vi "Read Numeric Text.vi"(9 "Digital in":refnum<class "Digital.lvclass">) -> (3 "Digital out":refnum<class "Digital.lvclass">, 4 "NumericText":refnum<class "NumericText.lvclass">)   [LabVIEW 2014, in "Raspberry Pi Compatible Compiler for LabVIEW.lvlib" / "Digital.lvclass"]
uses:
  Digital.lvclass
  NumericText/NumericText.lvclass
  Digital.lvclass/Digital.ctl
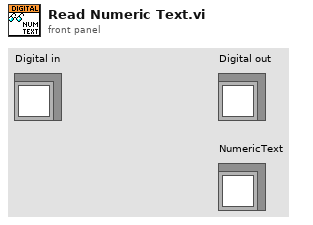
[diagram p1: front panel]
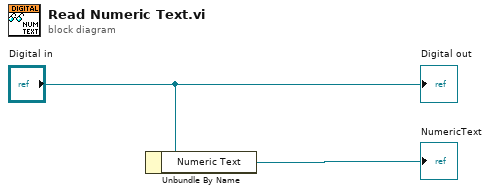
[diagram p0: block diagram]
diagram:
  n1 = Unbundle By Name("Digital in") -> ("Numeric Text"=→"NumericText":refnum<class "NumericText.lvclass">)
  "Digital out" <- "Digital in"
